vi "Initialize Engine Output.vi"(0 "Process in":refnum<class "Process.lvclass">, 1 "Init Data Buffers? (T)":bool=TRUE, 5 "Parameters":T2={"Interface Data"={"Name"="", "Unit ID"=0, "Refresh Rate"=0, "Write Rate"=0, "Write Mode"=enum."Value Change", "Interface Type"=enum."TCP Master", "TCP Settings"={"Address"="", "Port"=0, "Timeout"=0}, "Serial Settings"={"VISA resource name"="", "baud rate"=0, "parity (even)"=0, "flow control (none)"=0, "serial type"=enum."RTU", "Wire Mode"=-1}}, "Modbus Input Groups"=[], "Modbus Output Groups"=[], "error in (no error)"={"status"=FALSE, "code"=0, "source"=""}, "Modbus Input Engine Group Names"=[], "Modbus Output Engine Group Names"=[]} {"Interface Data"."Serial Settings"."Wire Mode" items=["Unknown"=-1, "RS485/Wire4"=0, "RS485/Wire2-EchoDTR"=1, "RS485/Wire2-CtrlDTR"=2, "RS485/Wire2-Auto"=3, "RS232/DTE"=128, "RS232/DCE"=129, "RS232/AUTO"=130]; "Interface Data"."Serial Settings"."parity (even)" items=["None", "Odd", "Even", "Mark", "Space"]; "Interface Data"."Serial Settings"."flow control (none)" items=["None", "XON/XOFF", "RTS/CTS", "XON/XOFF & RTS/CTS", "DTR/DSR", "XON/XOFF & DTR/DSR"]}, 11 "error in (no error)":errorcluster) -> (4 "Diagnostic Group Ref":T1, 6 "Output Group Refs":refnum<data-value>[](array[refnum]), 8 "Data Buffers":cluster{"Data":dbl[]}[](array[cluster]), 10 "Modbus Output Groups":T7[](array[typedef]), 15 "error out":errorcluster)   [LabVIEW 2021, in "Modbus Master Engine.lvlib"]
uses:
  Modbus Master Engine.lvlib
  <vilib>/NI/NIVS Inline Async API/_Data Access Engine/Access Type Classes/Read/Read.lvclass
  <vilib>/NI/NIVS Inline Async API/_VS Inline Async API/Process/Process.lvclass
  Bulk Data Access.ctl
  System Explorer/SubVIs/Modbus Type.ctl
  Shared/Controls/Data Model/Channel.ctl
  <vilib>/NI VeriStand/Custom Device API/Custom Device Channel Type.ctl
  Shared/Controls/Data Model/Mapping.ctl
  Shared/Controls/Data Model/DataType.ctl
  <vilib>/NI VeriStand/Custom Device API/Custom Device Item Ref.ctl
  Shared/Device Info.ctl
  Shared/Write Mode.ctl
  Shared/Controls/Interface Type.ctl
  Shared/Controls/Data Model/TCP Settings.ctl
  Shared/Controls/Data Model/Serial Settings.ctl
  <vilib>/NI/NIVS Inline Async API/_Data Access Engine/Data Access Engine/Types/Write.DVR.ctl
  <vilib>/NI/NIVS Inline Async API/_Data Access Engine/Access Type Classes/Write/Write.lvclass
  <vilib>/NI/NIVS Inline Async API/_VS Inline Async API/Process/Process.lvclass/Process.ctl
  <vilib>/NI/NIVS Inline Async API/_VS Inline Async API/Process/Data Member Access/Read Data Access.vi
  <vilib>/NI/NIVS Inline Async API/_Data Access Engine/Data Access Engine/Methods/Write.Lookup.vi
  <vilib>/NI/NIVS Inline Async API/_Data Access Engine/Data Access Engine/Data Access Engine.lvclass
  Shared/Modbus Master Shared.lvlib
  <vilib>/NI VeriStand/Custom Device API/Custom Device API.lvlib
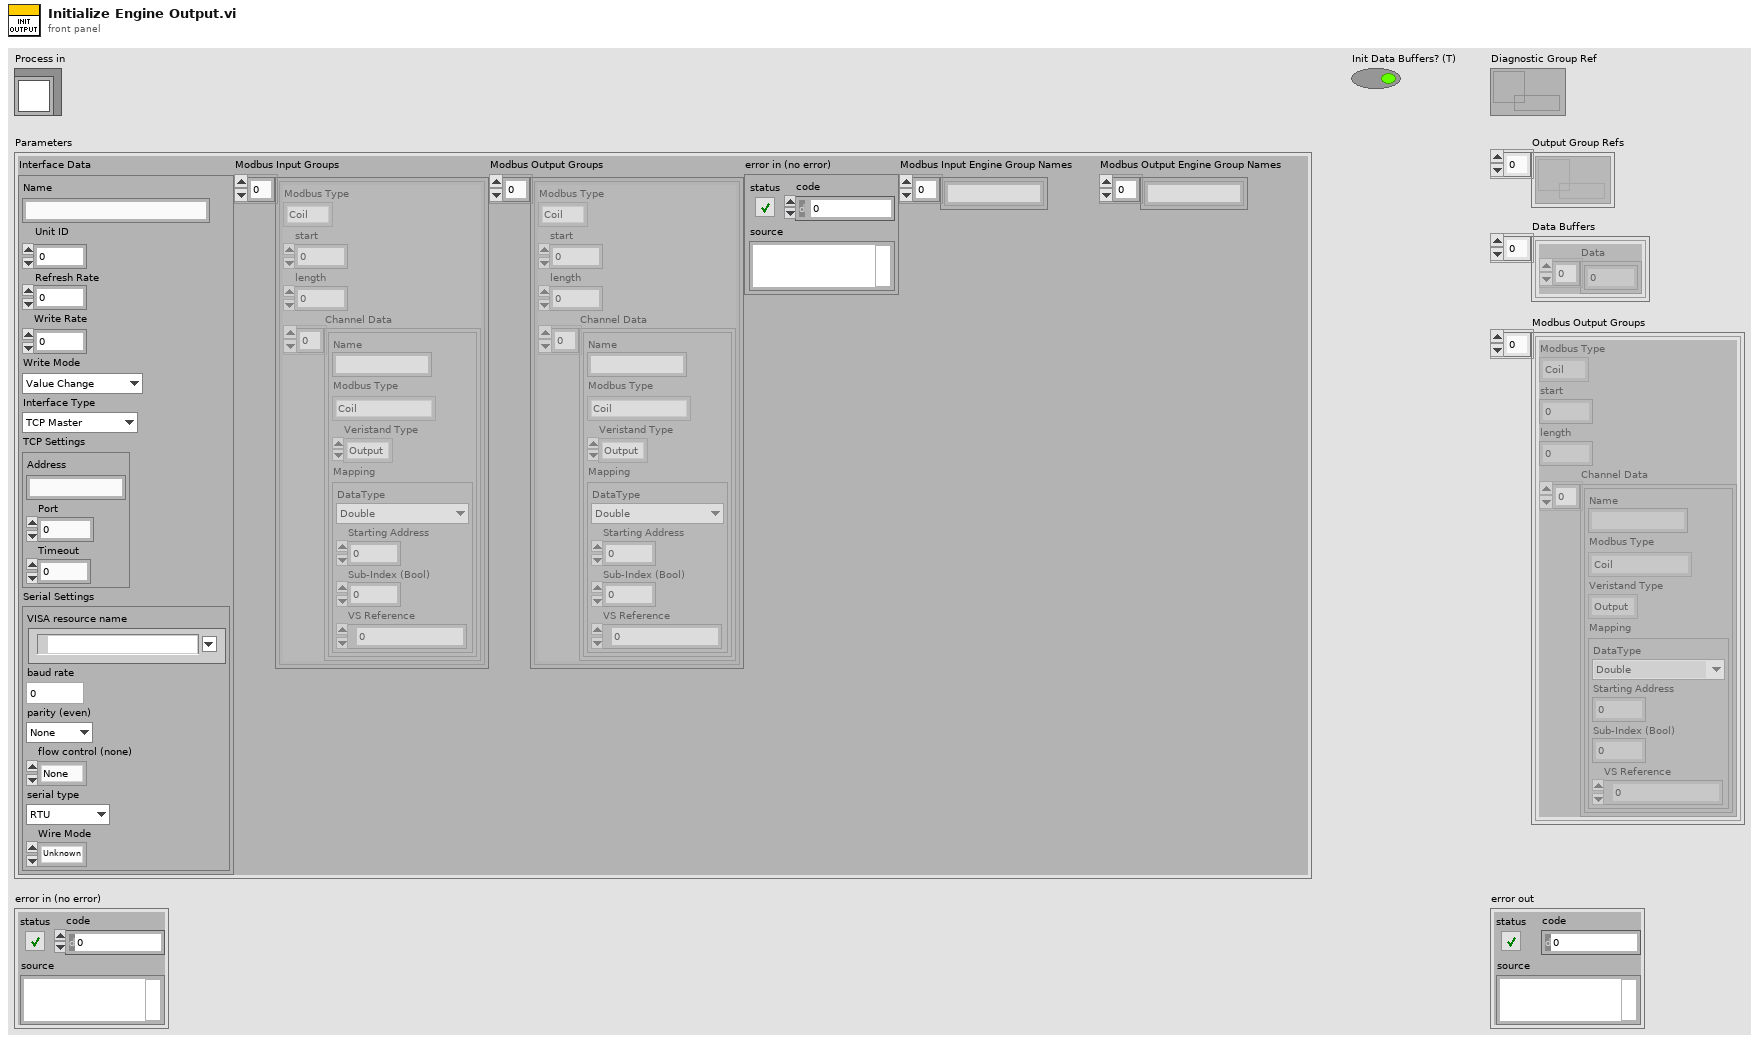
[diagram p1: front panel]
types:
  T1 = typedef "Data Access Engine.lvlib/Data Access Engine.lvclass/Write.DVR.ctl" = refnum<data-value>
  T2 = typedef "Modbus Master Shared.lvlib/Device Info.ctl" = cluster{"Interface Data":cluster{"Name":string, "Unit ID":u8, "Refresh Rate":i32, "Write Rate":i32, "Write Mode":T3, "Interface Type":T4, "TCP Settings":T5, "Serial Settings":T6}, "Modbus Input Groups":T7[], "Modbus Output Groups":T7[], "error in (no error)":errorcluster, "Modbus Input Engine Group Names":string[], "Modbus Output Engine Group Names":string[]}
  T3 = typedef "Modbus Master Shared.lvlib/Write Mode.ctl" = enum16{"Value Change", "Interval"}
  T4 = typedef "Modbus Master Shared.lvlib/Interface Type.ctl" = enum16{"TCP Master", "Serial Master", "TCP Slave", "Serial Slave"}
  T5 = typedef "Modbus Master Shared.lvlib/TCP Settings.ctl" = cluster{"Address":string, "Port":u16, "Timeout":i32}
  T6 = typedef "Modbus Master Shared.lvlib/Serial Settings.ctl" = cluster{"VISA resource name":refnum<visa-resource-name>, "baud rate":u32, "parity (even)":u16, "flow control (none)":u16, "serial type":enum16{"RTU", "ASCII"}, "Wire Mode":i16}
  T7 = typedef "Modbus Master Shared.lvlib/Bulk Data Access.ctl" = cluster{"Modbus Type":T8, "start":u16, "length":u16, "Channel Data":T9[]}
  T8 = typedef "Modbus Master Shared.lvlib/Modbus Type.ctl" = enum16{"Coil", "Discrete Input", "Holding Register", "Input Register"}
  T9 = typedef "Modbus Master Shared.lvlib/Channel.ctl" = cluster{"Name":string, "Modbus Type":T8, "Veristand Type":T10, "Mapping":T11}
  T10 = typedef "Custom Device API.lvlib/Custom Device Channel Type.ctl" = enum16{"Input", "Output"}
  T11 = typedef "Modbus Master Shared.lvlib/Mapping.ctl" = cluster{"DataType":T12, "Starting Address":u16, "Sub-Index (Bool)":u16, "VS Reference":T13}
  T12 = typedef "Modbus Master Shared.lvlib/DataType.ctl" = enum16{"Double", "Single", "I64", "I32", "I16", "I8", "U64", "U32", "U16", "U8", "Boolean"}
  T13 = typedef "Custom Device API.lvlib/Custom Device Item Ref.ctl" = u64
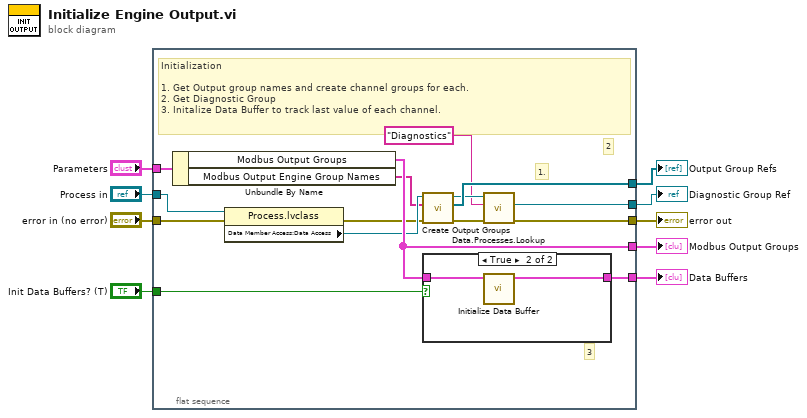
[diagram p0: block diagram]
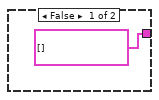
[diagram p2: hidden frame]
diagram:
  n1 = flat-sequence {
    tunnel: "Parameters" -> [w24]
    tunnel: [w23] -> w3
    tunnel: [w22] -> w4
    tunnel: "Process in" -> [w21]
    tunnel: [w18] -> w6
    tunnel: "error in (no error)" -> [w17]
    tunnel: [w13] -> w8
    tunnel: [w11] -> w9
    tunnel: "Init Data Buffers? (T)" -> [w10]
    frame #0 {
      # "3"
      # "2"
      # "1."
      # "Initialization\n\n1. Get Output group names and create channel groups for each.\n2. Get Diagnostic Group\n3. Initalize Data Buffer to track last value of each channel."
      n2 = Unbundle By Name(w24) -> ("Modbus Output Groups"=w23:T7[], "Modbus Output Engine Group Names"=w19:string[])
      n3 = property class="Process.lvclass"(reference=w21, error in=w17) -> (error out=w16:errorcluster, "Data Member Access:Data Access"=w20:refnum<class "Data Access Engine.lvclass">)  [unwired: 1 out]
      n4 = call "Create Output Groups.vi"("error in"=w16, "Input Engine Group Names"=w19, "Data Access Engine in"=w20) -> ("error out"=w12:errorcluster, "Array"=w18:refnum<data-value>[], "Data Access Engine out"=w15:refnum<class "Data Access Engine.lvclass">)  [unwired: 6 in]
      n5 = case shown="True" w10 {
        tunnel: w23 -> [_ w27]
        tunnel: [cluster{"Data":dbl[]}[] [] ("Data Buffers") w26] -> w22
        frame False {
        }
        frame True {
          n6 = call "Initialize Data Buffer.vi"("Output Groups"=w27) -> ("Data Buffers"=w26:cluster{"Data":dbl[]}[])  [unwired: 10 in]
        }
      }
      n7 = call-poly <vilib>:"Data.Processes.Lookup.vi"("error in (no error)"=w12, "Name"="Diagnostics", "Data Access API in"=w15) -> ("error out"=w11:errorcluster, "Ref"=w13:T1)  [unwired: 5 in, 2 out]
    }
  }
  "error out" <- w9
  "Output Group Refs" <- w6
  "Data Buffers" <- w4
  "Modbus Output Groups" <- w3
  "Diagnostic Group Ref" <- w8
